vi "Joystick and Camera XYZ.vi"() -> ()   [LabVIEW 2020]
uses:
  Classes/Controller/Camera/Machine Vision.ctl
  Classes/Controller/I-O/I-O.lvclass
  Classes/Controller/Motion/Motion.lvclass
  Classes/Controller/Camera/Camera.lvclass
  Classes/Controller/Controller.lvclass
  Classes/Controller/Motion/A3200/A3200.lvclass
panel:
  out "XYZTheta Out":dbl[](array[numeric])
  in  "Machine Vision":T1
  in  "Move 10cm Right":bool
  in  "Move 10cm Backward":bool
  in  "Move 10cm Forward":bool
  in  "Move 10cm Left":bool
  in  "Record Measurement":bool=TRUE
  in  "Dismount Silicon Tray":bool
  in  "Secure Silicon Tray":bool
  in  "Z Go":bool
  in  "Position":dbl
  in  "XYZTheta":dbl[](array[numeric])
  in  "Go":bool
  in  "Joystick":bool
  out "Sum":dbl[](array[numeric])
  out "Gantry":dbl[](array[numeric])
  in  "Stop":bool
  out "Image":T2(plugin-control)
  out "Camera":dbl[](array[numeric])
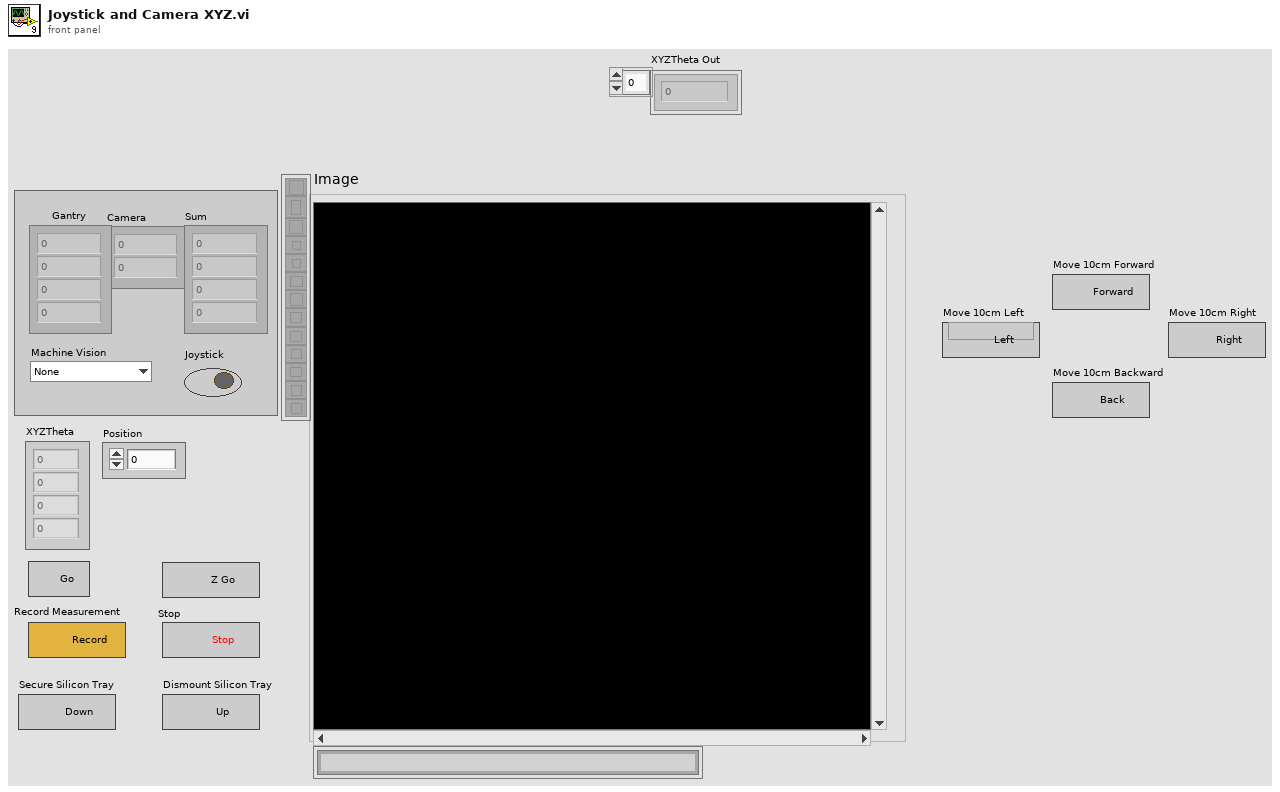
[diagram p1: front panel]
types:
  T1 = typedef "Camera.lvclass/Machine Vision.ctl" = enum16{"None", "Tray Fiducials", "HPK Silicon", "Hexaboard", "Corner (TL, BR)", "Corner (BL, TR)"}
  T2 = typedef "IMAQ Image.ctl" = refnum<image>
  T3 = enum16{"open", "replace", "create", "open or create", "replace or create", "replace or create with confirmation"}
  T4 = typedef "Controller.lvclass/Controllers.ctl" = cluster{"I-O.lvclass":refnum<class "I-O.lvclass">, "Dispenser.lvclass":refnum<class "Dispenser.lvclass">, "Gantry":refnum<k24>}
  T5 = typedef "I-O.lvclass/Pin Map.ctl" = cluster{"Region Valves":i32[], "Extra Valves":dbl[][][], "Tool Primary Valve":i32, "Tool Secondary Valve":i32, "Region Sensors":i32[], "Extra Sensors":dbl[][][], "Tool Primary Sensor":dbl, "Tool Secondary Sensor":dbl, "Compression Sensor":dbl, "5V":i32}
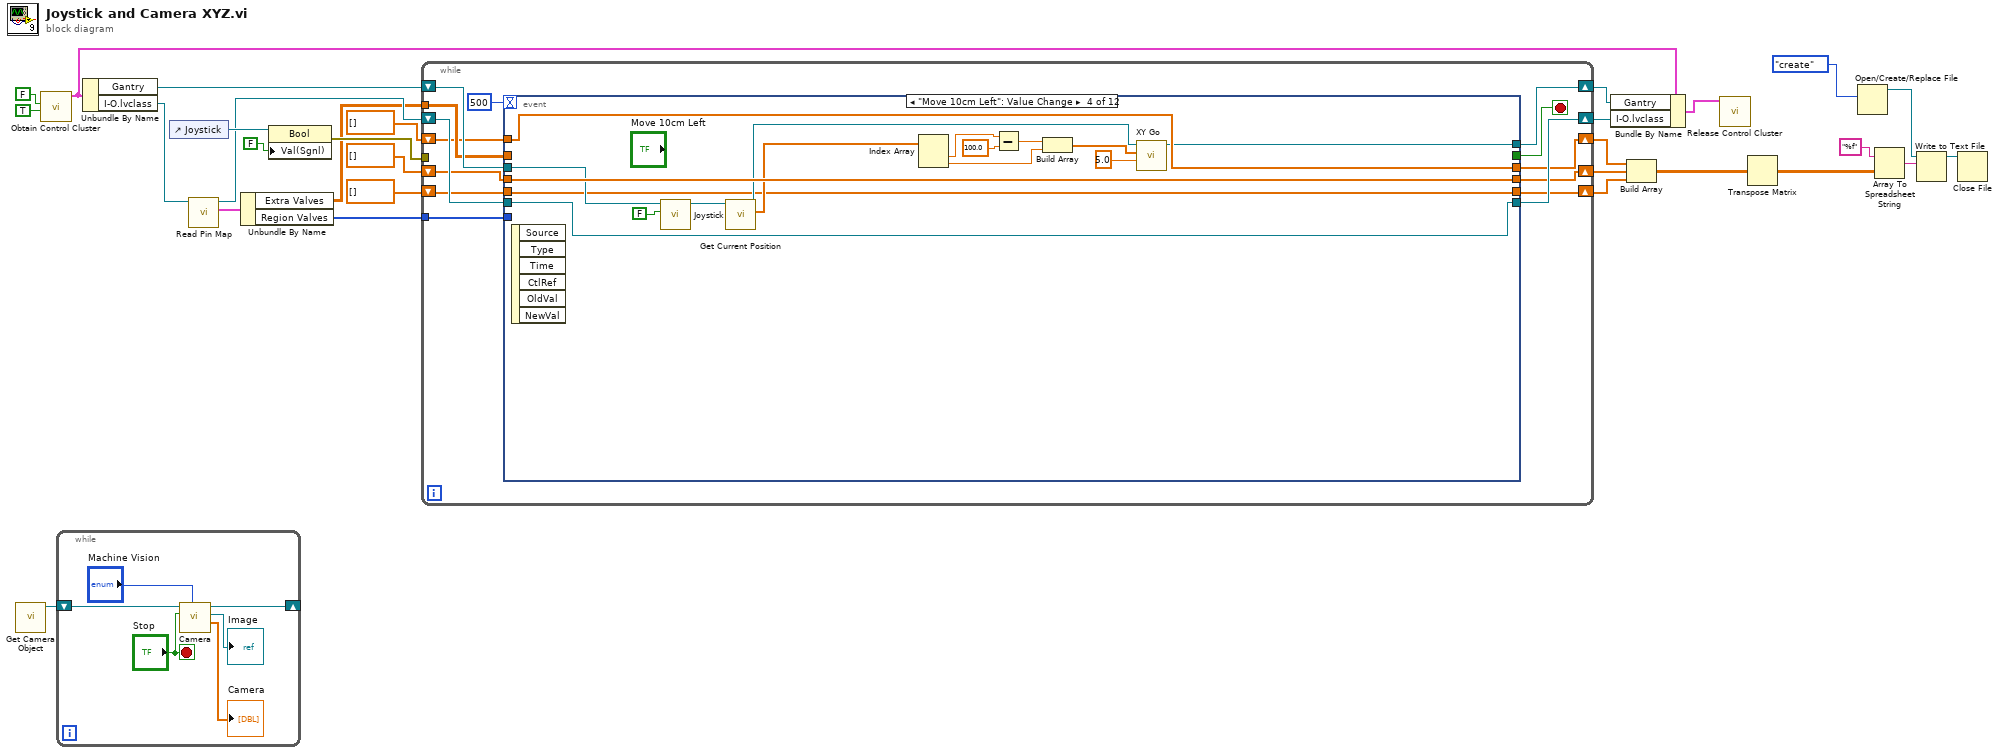
[diagram p0: block diagram]
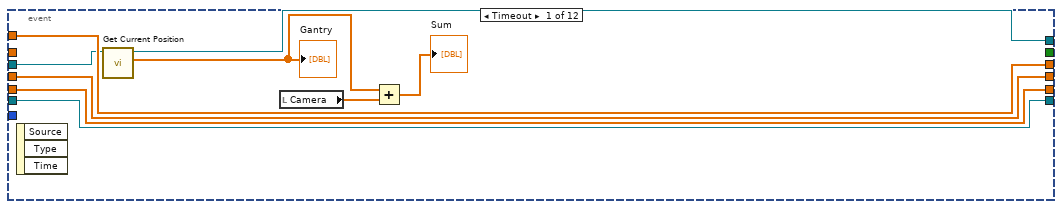
[diagram p2: hidden frame]
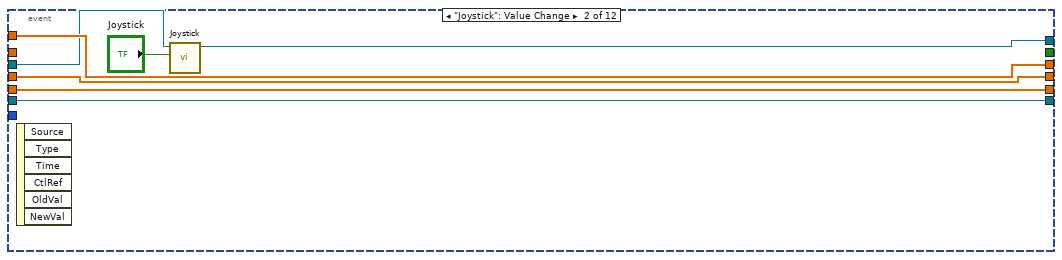
[diagram p3: hidden frame]
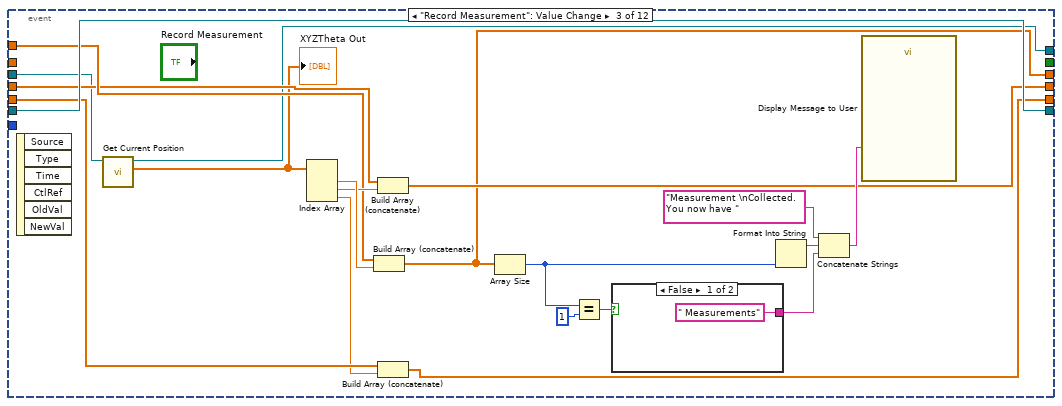
[diagram p4: hidden frame]
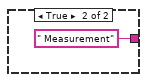
[diagram p5: hidden frame]
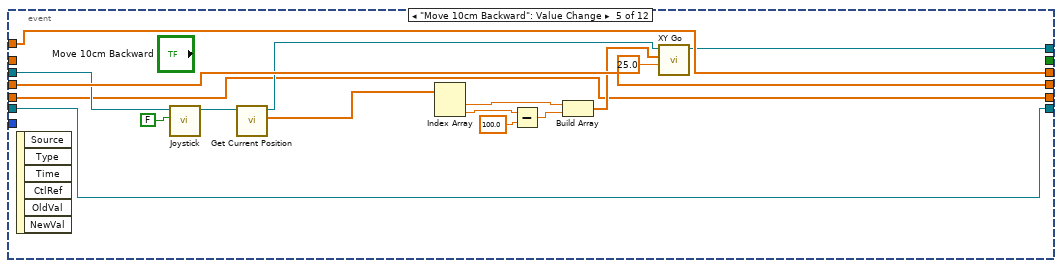
[diagram p6: hidden frame]
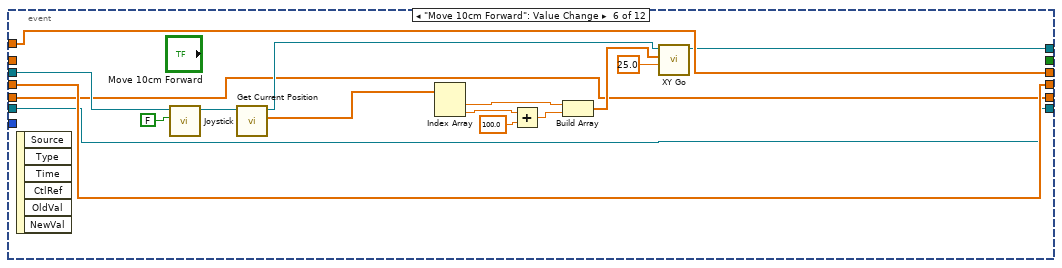
[diagram p7: hidden frame]
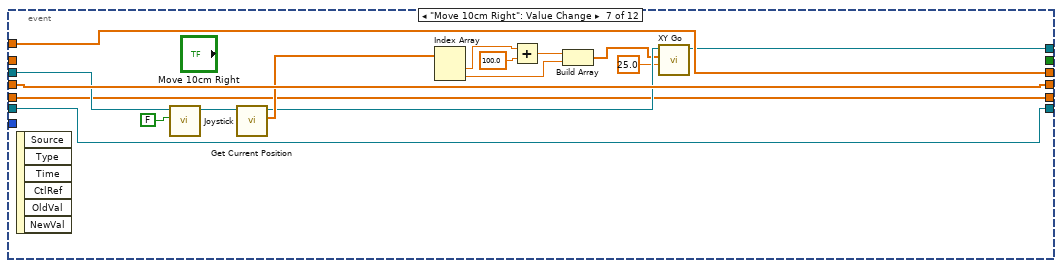
[diagram p8: hidden frame]
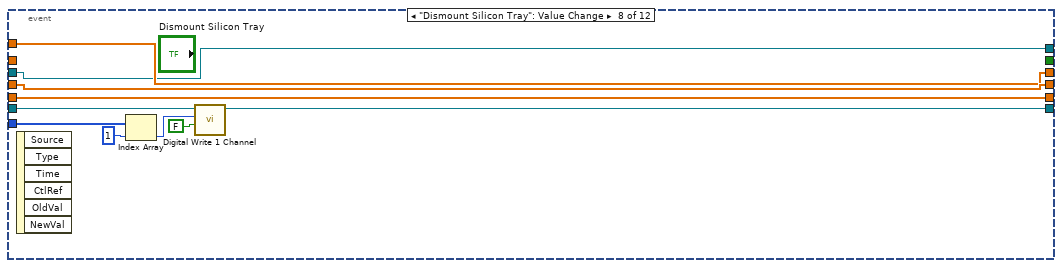
[diagram p9: hidden frame]
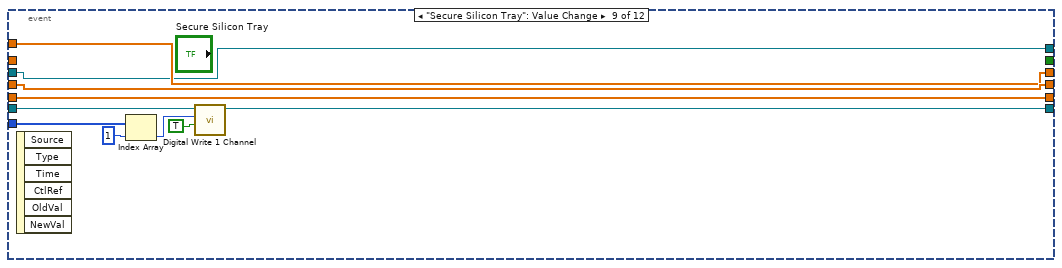
[diagram p10: hidden frame]
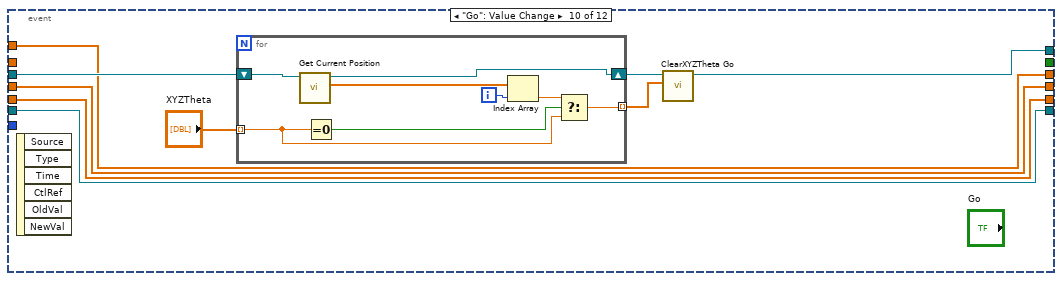
[diagram p11: hidden frame]
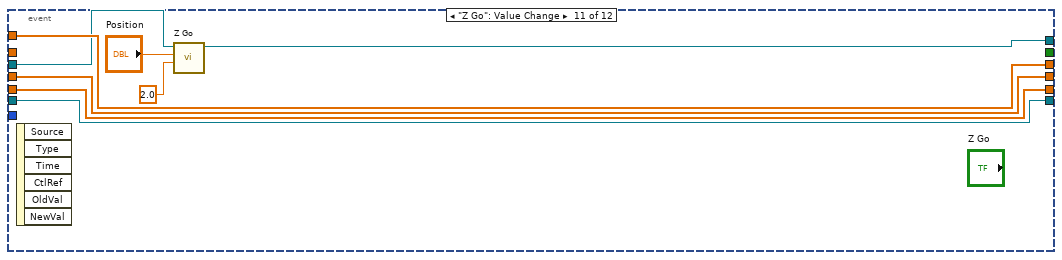
[diagram p12: hidden frame]
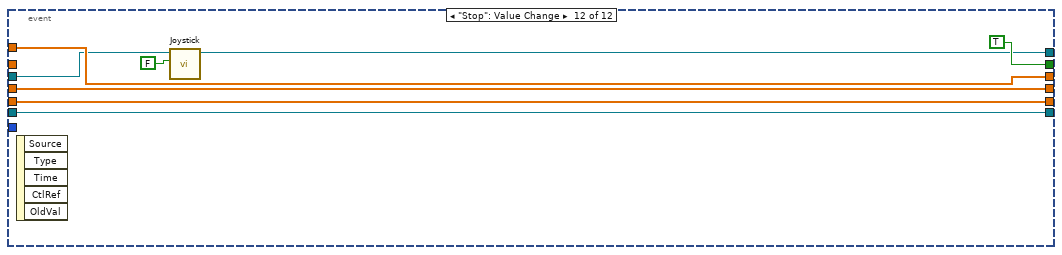
[diagram p13: hidden frame]
diagram:
  n1 = call "Get Camera Object.vi"() -> ("Camera out"=w23:refnum<class "Camera.lvclass">)  [unwired: 10 in, 1 out]
  n2 = call "Obtain Control Cluster.vi"("I/O"=TRUE, "Dispense"=FALSE) -> ("Control Out"=w3:T4)  [unwired: 9 in]
  n3 = while {
    shift-right: [w34] -> _
    shift-left: w23 -> [w35]
    stop <- "Stop" stop-if-true
    n4 = call "Camera.vi"("Machine Vision"="Machine Vision", "Stop"="Stop", "Camera in"=w35) -> ("Camera"=→"Camera":dbl[], "Image"=→"Image":T2, "Camera out"=w34:refnum<class "Camera.lvclass">)  [unwired: 5 in, 1 out]
  }
  n5 = Unbundle By Name(w3) -> ("Gantry"=w24:refnum<k24>, "I-O.lvclass"=w22:refnum<class "I-O.lvclass">)
  n6 = control-ref of="Joystick"() -> (w28:refnum<vi>)
  n7 = call-dynamic "Read Pin Map.vi"("I-O in"=w22) -> ("Pin Map 2"=w20:T5, "I-O out"=w21:refnum<class "I-O.lvclass">)  [unwired: 8 in, 1 out]
  n8 = Unbundle By Name(w20) -> ("Extra Valves"=w18:dbl[][][], "Region Valves"=w19:i32[])
  n9 = property class="Bool"(reference=w28, "Val(Sgnl)"=FALSE ("Value (Signaling)")) -> (error out=w27:errorcluster)  [unwired: 1 in, 1 out]
  n10 = while {
    shift-right: [w38] -> w4
    shift-left: w24 -> [w47]
    tunnel: w27 -> [_]
    shift-right: [w45] -> w2
    shift-left: w21 -> [w46]
    tunnel: w19 -> [w44]
    tunnel: w18 -> [w43]
    shift-right: [w40] -> w7
    shift-left: dbl[] [] -> [w42]
    shift-right: [w39] -> w8
    shift-left: dbl[] [] -> [w41]
    shift-right: [w37] -> w5
    shift-left: dbl[] [] -> [w36]
    stop <- w48 stop-if-true
    n11 = event shown="[3] \"Move 10cm Left\": Value Change" {
      selector: _ -> [_ _ _ _ _ _ _ _ _ _ _ _]
      dyn-events: _ -> [_ _ _ _ _ _ _ _ _ _ _ _]
      timeout: 500 -> [_ _ _ _ _ _ _ _ _ _ _ _]
      tunnel: [_ _ _ _ _ _ _ _ _ _ _ TRUE] -> w48
      tunnel: w47 -> [w52 w60 w71 w91 w106 w124 w138 w153 w163 w179 w193 w199]
      tunnel: w46 -> [w56 w65 w85 w88 w104 w120 w136 w159 w171 w176 w196 w203]
      tunnel: [w56 w65 w85 w88 w104 w120 w136 w156 w166 w176 w196 w203] -> w45
      tunnel: w44 -> [_ _ _ _ _ _ _ w161 w170 _ _ _]
      tunnel: w43 -> [_ _ _ _ _ _ _ _ _ _ _ _]
      tunnel: w42 -> [w55 w64 w72 w99 w115 w131 w147 w155 w165 w175 w195 w202]
      tunnel: [w55 w64 w76 w99 w115 w131 w147 w155 w165 w175 w195 w202] -> w40
      tunnel: w41 -> [w54 w63 w73 w98 w114 w130 w146 w154 w164 w174 w194 w201]
      tunnel: [w54 w63 w75 w98 w114 w130 w146 w154 w164 w174 w194 w201] -> w39
      tunnel: [w51 w61 w69 w90 w107 w122 w139 w153 w163 w173 w190 w198] -> w38
      tunnel: [w50 w59 w66 w89 w105 w121 w137 w152 w162 w172 w189 w197] -> w37
      tunnel: w36 -> [w50 w59 w68 w89 w105 w121 w137 w152 w162 w172 w189 w197]
      event Timeout {
        n12 = event-data() -> ()  [unwired: 1 in, 3 out]
        n13 = call "Get Current Position.vi"("Gantry 2"=w52) -> ("XYZTheta Out"=w53:dbl[], "Gantry 3"=w51:refnum<k24>)  [unwired: 8 in, 1 out]
        "Gantry" <- w53
        n14 = local read "Camera"() -> (w58:dbl[])
        n15 = Add(x=w53, y=w58) -> (x+y=→"Sum":dbl[])
      }
      event "Joystick": Value Change {
        n16 = event-data() -> ()  [unwired: 1 in, 6 out]
        n17 = call "Joystick.vi"("Joystick"="Joystick", "Gantry 2"=w60) -> ("Gantry 3"=w61:refnum<k24>)  [unwired: 8 in, 1 out]
      }
      event "Record Measurement": Value Change {
        n18 = event-data() -> ()  [unwired: 1 in, 6 out]
        n19 = call "Get Current Position.vi"("Gantry 2"=w71) -> ("XYZTheta Out"=w70:dbl[], "Gantry 3"=w69:refnum<k24>)  [unwired: 8 in, 1 out]
        "XYZTheta Out" <- w70
        n20 = Index Array(array=w70) -> (element #1=w84:dbl, element #2=w74:dbl, element #3=w67:dbl)  [unwired: 3 in]
        n21 = Build Array (concatenate) "Build Array"(w73, w84) -> (w75:dbl[])
        n22 = Build Array (concatenate)(w72, w74) -> (w76:dbl[])
        n23 = Build Array (concatenate)(w68, w67) -> (w66:dbl[])
        n24 = Array Size(array=w75) -> (size(s)=w79:i32)
        n25 = Equal?(x=w79, y=1) -> (x = y?=w78:bool)
        n26 = case shown="False" w78 {
          tunnel: [" Measurements" " Measurement"] -> w77
          frame False {
          }
          frame True {
          }
        }
        n27 = Format Into String(w79) -> (resulting string=w83:string)  [unwired: 3 in, 1 out]
        n28 = Concatenate Strings("Measurement \nCollected. You now have ", w83, w77) -> (w81:string)
        n29 = call "Display Message to User"("Message"=w81) -> ()  [unwired: 9 in, 2 out]
      }
      event "Move 10cm Left": Value Change {
        n30 = event-data() -> ()  [unwired: 1 in, 6 out]
        n31 = call "Joystick.vi"("Joystick"=FALSE, "Gantry 2"=w91) -> ("Gantry 3"=w96:refnum<k24>)  [unwired: 8 in, 1 out]
        n32 = call "Get Current Position.vi"("Gantry 2"=w96) -> ("XYZTheta Out"=w92:dbl[], "Gantry 3"=w93:refnum<k24>)  [unwired: 8 in, 1 out]
        n33 = Index Array(array=w92) -> (element #1=w103:dbl, element #2=w100:dbl)  [unwired: 2 in]
        n34 = Subtract(x=w103, y=100.0) -> (x-y=w101:dbl)
        n35 = Build Array(w101, w100) -> (w94:dbl[])
        n36 = call "XY Go.vi"("Speed"=5.0, "XY"=w94, "Gantry 2"=w93) -> ("Gantry 3"=w90:refnum<k24>)  [unwired: 7 in, 1 out]
      }
      event "Move 10cm Backward": Value Change {
        n37 = event-data() -> ()  [unwired: 1 in, 6 out]
        n38 = call "Joystick.vi"("Joystick"=FALSE, "Gantry 2"=w106) -> ("Gantry 3"=w112:refnum<k24>)  [unwired: 8 in, 1 out]
        n39 = call "Get Current Position.vi"("Gantry 2"=w112) -> ("XYZTheta Out"=w111:dbl[], "Gantry 3"=w110:refnum<k24>)  [unwired: 8 in, 1 out]
        n40 = Index Array(array=w111) -> (element #1=w116:dbl, element #2=w119:dbl)  [unwired: 2 in]
        n41 = Subtract(x=w119, y=100.0) -> (x-y=w117:dbl)
        n42 = Build Array(w116, w117) -> (w108:dbl[])
        n43 = call "XY Go.vi"("Speed"=25.0, "XY"=w108, "Gantry 2"=w110) -> ("Gantry 3"=w107:refnum<k24>)  [unwired: 7 in, 1 out]
      }
      event "Move 10cm Forward": Value Change {
        n44 = event-data() -> ()  [unwired: 1 in, 6 out]
        n45 = call "Joystick.vi"("Joystick"=FALSE, "Gantry 2"=w124) -> ("Gantry 3"=w128:refnum<k24>)  [unwired: 8 in, 1 out]
        n46 = call "Get Current Position.vi"("Gantry 2"=w128) -> ("XYZTheta Out"=w127:dbl[], "Gantry 3"=w123:refnum<k24>)  [unwired: 8 in, 1 out]
        n47 = Index Array(array=w127) -> (element #1=w133:dbl, element #2=w134:dbl)  [unwired: 2 in]
        n48 = Add(x=w134, y=100.0) -> (x+y=w132:dbl)
        n49 = Build Array(w133, w132) -> (w126:dbl[])
        n50 = call "XY Go.vi"("Speed"=25.0, "XY"=w126, "Gantry 2"=w123) -> ("Gantry 3"=w122:refnum<k24>)  [unwired: 7 in, 1 out]
      }
      event "Move 10cm Right": Value Change {
        n51 = event-data() -> ()  [unwired: 1 in, 6 out]
        n52 = call "Joystick.vi"("Joystick"=FALSE, "Gantry 2"=w138) -> ("Gantry 3"=w144:refnum<k24>)  [unwired: 8 in, 1 out]
        n53 = call "Get Current Position.vi"("Gantry 2"=w144) -> ("XYZTheta Out"=w143:dbl[], "Gantry 3"=w142:refnum<k24>)  [unwired: 8 in, 1 out]
        n54 = Index Array(array=w143) -> (element #1=w148:dbl, element #2=w149:dbl)  [unwired: 2 in]
        n55 = Add(x=w148, y=100.0) -> (x+y=w150:dbl)
        n56 = Build Array(w150, w149) -> (w140:dbl[])
        n57 = call "XY Go.vi"("Speed"=25.0, "XY"=w140, "Gantry 2"=w142) -> ("Gantry 3"=w139:refnum<k24>)  [unwired: 7 in, 1 out]
      }
      event "Dismount Silicon Tray": Value Change {
        n58 = event-data() -> ()  [unwired: 1 in, 6 out]
        n59 = Index Array(array=w161, index=1) -> (element=w158:i32)
        n60 = call-dynamic "Digital Write 1 Channel.vi"("Value"=FALSE, "Channel"=w158, "I-O.lvclass"=w159) -> ("I-O.lvclass 2"=w156:refnum<class "I-O.lvclass">)  [unwired: 7 in, 1 out]
      }
      event "Secure Silicon Tray": Value Change {
        n61 = event-data() -> ()  [unwired: 1 in, 6 out]
        n62 = Index Array(array=w170, index=1) -> (element=w168:i32)
        n63 = call-dynamic "Digital Write 1 Channel.vi"("Value"=TRUE, "Channel"=w168, "I-O.lvclass"=w171) -> ("I-O.lvclass 2"=w166:refnum<class "I-O.lvclass">)  [unwired: 7 in, 1 out]
      }
      event "Go": Value Change {
        n64 = event-data() -> ()  [unwired: 1 in, 6 out]
        n65 = for {
          tunnel: "XYZTheta" -> [w186] mode=indexing
          tunnel: [w184] -> w178 mode=indexing
          shift-right: [w181] -> w177
          shift-left: w179 -> [w182]
          i -> [w188]
          n66 = call "Get Current Position.vi"("Gantry 2"=w182) -> ("XYZTheta Out"=w183:dbl[], "Gantry 3"=w181:refnum<k24>)  [unwired: 8 in, 1 out]
          n67 = Equal To 0?(x=w186) -> (x = 0?=w187:bool)
          n68 = Index Array(array=w183, index=w188) -> (element=w185:dbl)
          n69 = Select(t=w185, s=w187, f=w186) -> (s? t:f=w184:dbl)
        }
        n70 = call "ClearXYZTheta Go.vi"("XYZTheta In"=w178, "Gantry 2"=w177) -> ("Gantry 3"=w173:refnum<k24>)  [unwired: 7 in, 2 out]
      }
      event "Z Go": Value Change {
        n71 = event-data() -> ()  [unwired: 1 in, 6 out]
        n72 = call "Z Go.vi"("Speed"=2.0, "Position"="Position", "Gantry"=w193) -> ("Gantry"=w190:refnum<k24>)  [unwired: 7 in, 1 out]
      }
      event "Stop": Value Change {
        n73 = event-data() -> ()  [unwired: 1 in, 5 out]
        n74 = call "Joystick.vi"("Joystick"=FALSE, "Gantry 2"=w199) -> ("Gantry 3"=w198:refnum<k24>)  [unwired: 8 in, 1 out]
      }
    }
  }
  n75 = Bundle By Name(cluster=w3, "Gantry"=w4, "I-O.lvclass"=w2) -> (w1:T4)
  n76 = Build Array(w8, w7, w5) -> (w10:dbl[][])
  n77 = call "Release Control Cluster.vi"("output cluster"=w1) -> ()  [unwired: 11 in]
  n78 = Transpose Matrix(1:w10) -> (0:w9:dbl[][])
  n79 = Open/Create/Replace File(operation (0:open)=T3."create") -> (refnum out=w14:refnum<file>)  [unwired: 5 in, 2 out]
  n80 = Array To Spreadsheet String(array=w9, 3:"%f" ("format string")) -> (spreadsheet string=w12:string)  [unwired: 1 in]
  n81 = Write to Text File(file (use dialog)=w14, text=w12) -> (refnum out=w11:refnum<file>)  [unwired: 2 in, 2 out]
  n82 = Close File(refnum=w11) -> ()  [unwired: 1 in, 2 out]
